vi "DeserializeInitObjectStack.vi"(8 "error in (no error)":errorcluster, 9 "ClassName Cache":refnum<data-value>, 10 "SerializableDataOverride (parent, child)":variant[](array[variant]), 11 "Target Object":refnum<class "BlueSerializable.lvclass">) -> (0 "error out":errorcluster, 2 "Object stack (child, parent)":T1[](array[typedef]), 3 "Target Object (dup)":refnum<class "BlueSerializable.lvclass">)   [LabVIEW 2020, in "BlueSerialization.lvlib" / "BlueSerializer.lvclass"]
uses:
  BlueSerializer.lvclass
  Support/SetSerializableDataObject.ctl
  BlueSerializable/BlueSerializable.lvclass
  ClassNameCacheCluster.ctl
  ClassNameCacheMap.ctl
  ClassNameObj.ctl
  Support/GetParentClassesHiererchy.vi
  ClassNameCacheWrite.vi
  LVOOP Get Default Object Inline.vi
  GetDescendantType.vi
  LVOOP is Same or Descendant Class Inline.vi
  <vilib>/Utility/LVClass/Get LV Class Name.vi
  GetClassListInMemory.vi
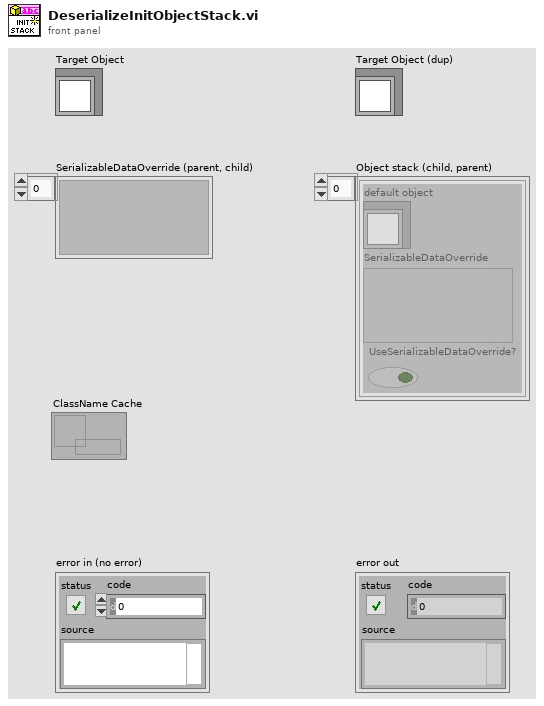
[diagram p1: front panel]
types:
  T1 = typedef "BlueSerialization.lvlib/BlueSerializer.lvclass/SetSerializableDataObject.ctl" = cluster{"default object":refnum<class "BlueSerializable.lvclass">, "SerializableDataOverride":variant, "UseSerializableDataOverride?":bool}
  T2 = typedef "BlueSerialization.lvlib/BlueSerializer.lvclass/ClassNameObj.ctl" = cluster{"class name":string, "default object":refnum<class>}
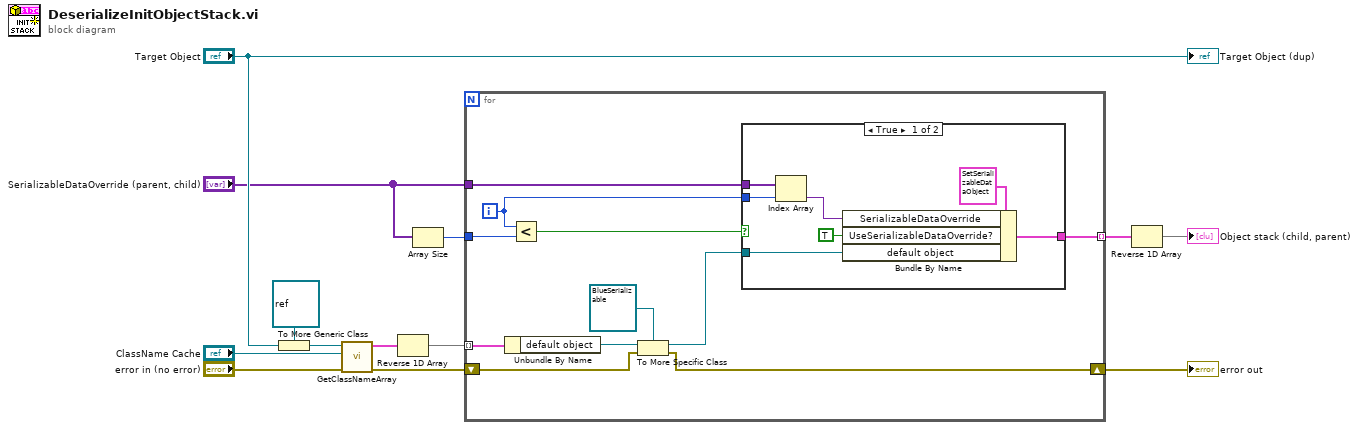
[diagram p0: block diagram]
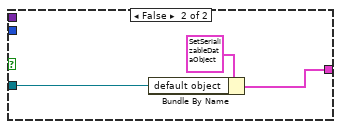
[diagram p2: hidden frame]
diagram:
  n1 = To More Generic Class(target class=refnum<class> refnum ("LabVIEW Object"), reference="Target Object") -> (generic class reference=w10:refnum<class>)
  n2 = call "GetClassNameArray.vi"("error in (no error)"="error in (no error)", "ClassName Cache"="ClassName Cache", "LabVIEW Object in"=w10) -> ("error out"=w13:errorcluster, "Class (child,parent)"=w8:T2[])  [unwired: 7 in]
  n3 = Reverse 1D Array(array=w8) -> (reversed array=w7:T2[])
  n4 = Array Size(array="SerializableDataOverride (parent, child)") -> (size(s)=w6:i32)
  n5 = for {
    tunnel: w7 -> [w24] mode=indexing
    shift-right: [w20] -> w1
    shift-left: w13 -> [w21]
    tunnel: w6 -> [w18]
    tunnel: "SerializableDataOverride (parent, child)" -> [w17]
    tunnel: [w15] -> w4 mode=indexing
    i -> [w14]
    n6 = Unbundle By Name(w24) -> ("default object"=w22:refnum<class>)
    n7 = Less?(x=w14, y=w18) -> (x < y?=w16:bool)
    n8 = To More Specific Class(target class=refnum<class "BlueSerializable.lvclass"> refnum ("BlueSerializer.lvlib:BlueSerializable.lvclass"), reference=w22, error in=w21) -> (specific class reference=w19:refnum<class "BlueSerializable.lvclass">, error out=w20:errorcluster)
    n9 = case shown="True" w16 {
      tunnel: w19 -> [w30 w33]
      tunnel: w17 -> [w29 _]
      tunnel: [w26 w32] -> w15
      tunnel: w14 -> [w25 _]
      frame True {
        n10 = Index Array(array=w29, index=w25) -> (element=w28:variant)
        n11 = Bundle By Name(cluster=T1 {"default object"=refnum, "SerializableDataOverride"=variant, "UseSerializableDataOverride?"=FALSE} ("Cluster"), "SerializableDataOverride"=w28, "UseSerializableDataOverride?"=TRUE, "default object"=w30) -> (w26:T1)
      }
      frame False {
        n12 = Bundle By Name(cluster=T1 {"default object"=refnum, "SerializableDataOverride"=variant, "UseSerializableDataOverride?"=FALSE} ("Cluster"), "default object"=w33) -> (w32:T1)
      }
    }
  }
  "error out" <- w1
  n13 = Reverse 1D Array(array=w4) -> (reversed array=→"Object stack (child, parent)":T1[])
  "Target Object (dup)" <- "Target Object"
